vi "Popup.vi"(8 "error in (no error)":errorcluster, 9 "Panel":refnum<class "Panel.lvclass">, 10 "String in":string, 11 "Generic Data Type in":refnum<class "Generic Data Type.lvclass">) -> (0 "error out":errorcluster, 2 "String out":string, 3 "Generic Data Type out":refnum<class "Generic Data Type.lvclass">)   [LabVIEW 2018, in "Generic Data Type.lvclass"]
uses:
  Generic Data Type.lvclass
  <vilib>/MGI/Panel Manager/Panel/Panel/Panel.lvclass
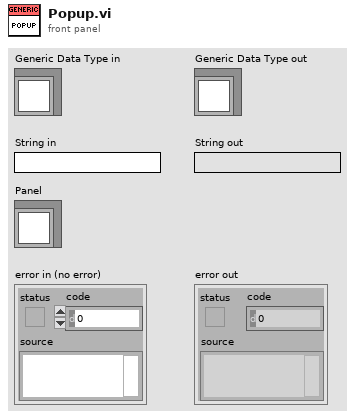
[diagram p1: front panel]
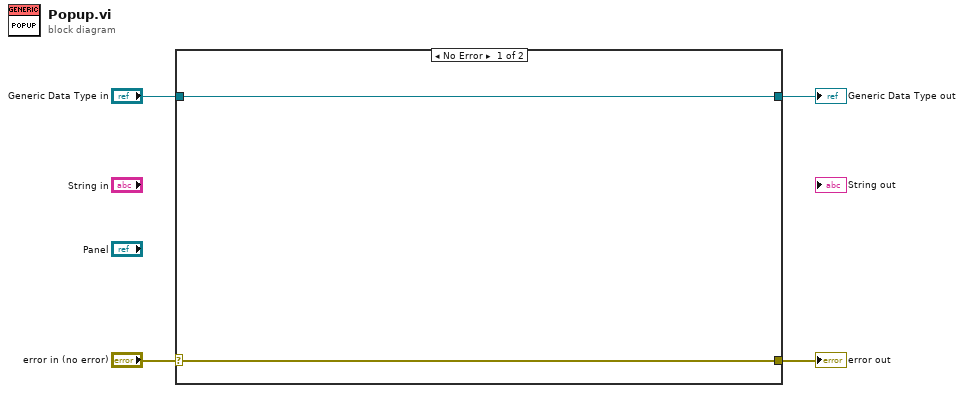
[diagram p0: block diagram]
diagram:
  n1 = case shown="No Error" "error in (no error)" {
    selector: "error in (no error)" -> [w5 w8]
    tunnel: [w5 w8] -> w3
    tunnel: [w6 w7] -> w1
    tunnel: "Generic Data Type in" -> [w6 w7]
    frame No Error {
    }
    frame Error {
    }
  }
  "error out" <- w3
  "Generic Data Type out" <- w1
